vi "template.vi"() -> ()   [LabVIEW 2023]
uses:
  states.ctl
panel:
  in  "Stop Receiving GPS Data":bool
  in  "Stop Receiving Safety Data":bool
  in  "Start":bool
  in  "Stop":bool
  in  "Speed Threshold (km/h)":dbl
  out "Arm System":bool
  out "Laser 2":bool
  out "Laser 1":bool
  out "Safety System 2":bool[](array[boolean])
  out "Safety System 1":bool[](array[boolean])
  out "GPS":cluster{"Lat":dbl, "Lon":dbl, "Speed":dbl} {"Lon" format="%#_15g"; "Lat" format="%#_16g"}
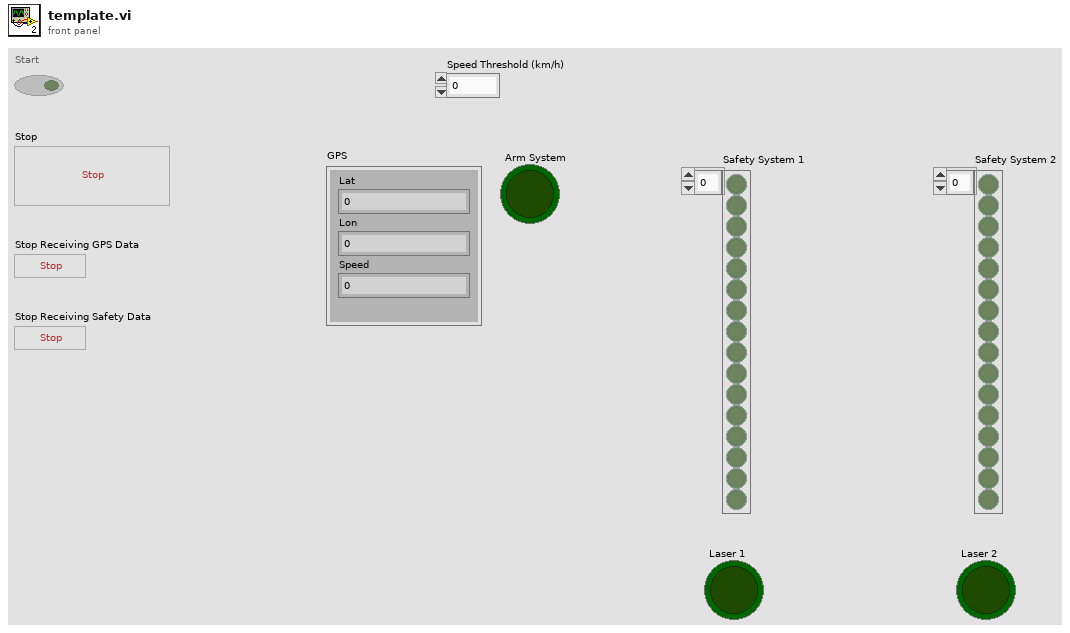
[diagram p1: front panel]
types:
  T1 = typedef "states.ctl" = enum16{"Set Speed Threshold", "Wait for Start", "Wait for TCP", "Main Loop"}
  T2 = enum8{"Enabled", "Disabled", "Disabled and Grayed Out"}
  T3 = enum16{"Standard", "Buffered", "CRLF", "Immediate"}
  T4 = cluster{"Latitude":dbl, "Longitude":dbl, "speed":dbl}
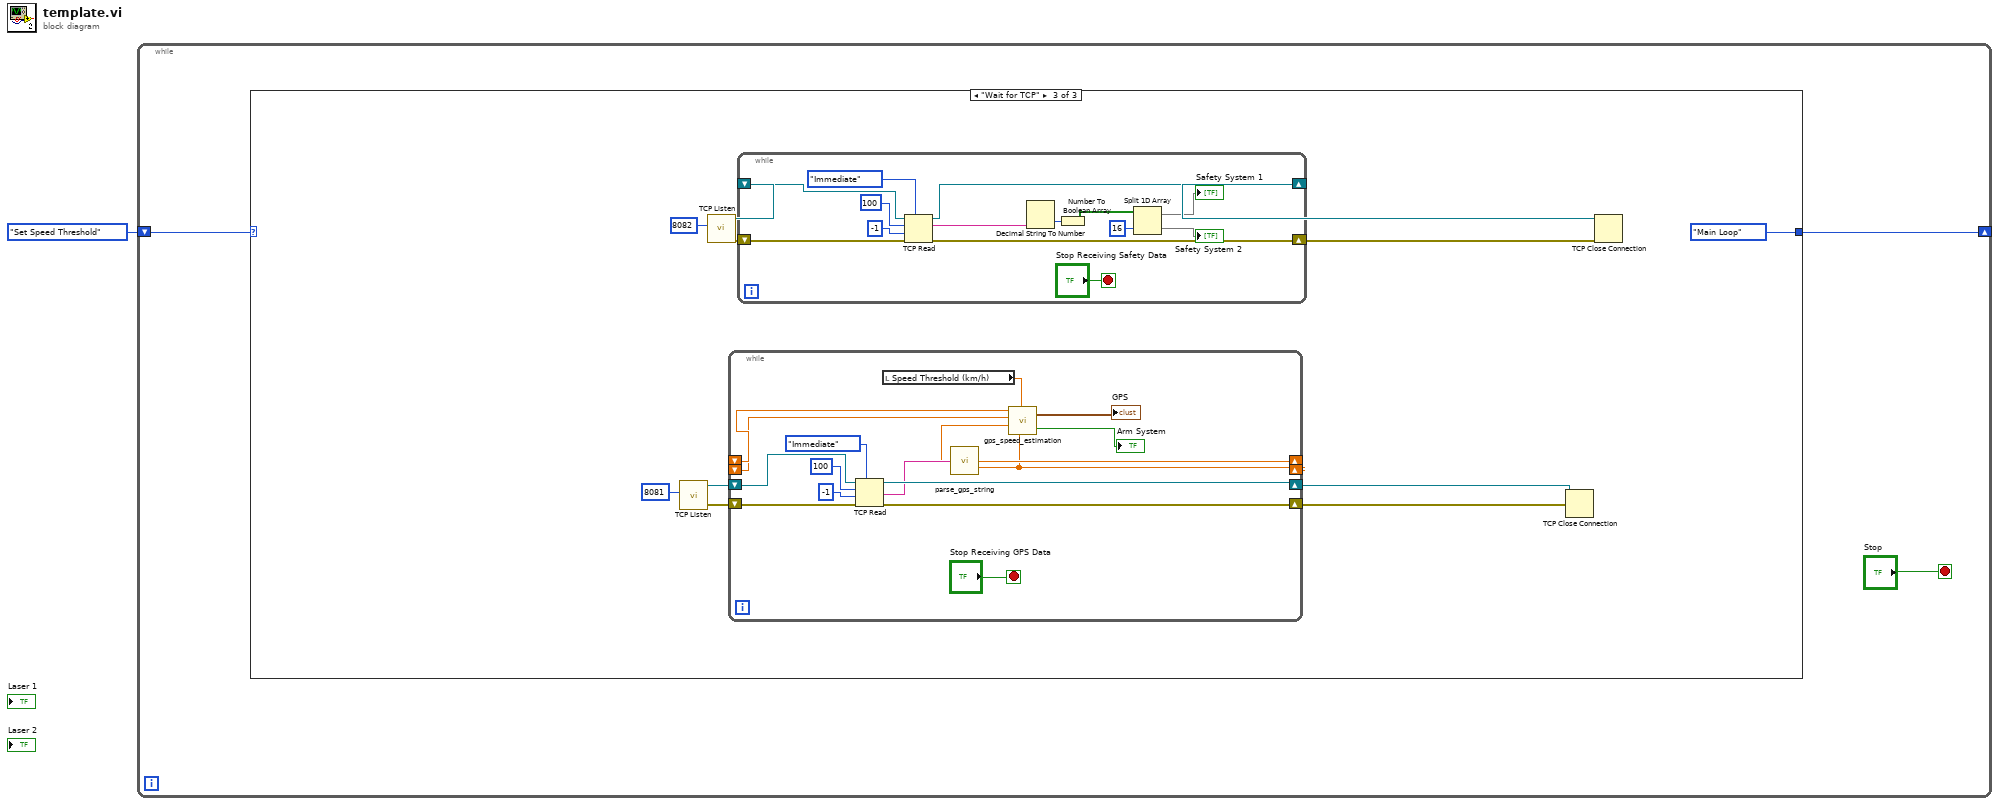
[diagram p0: block diagram]
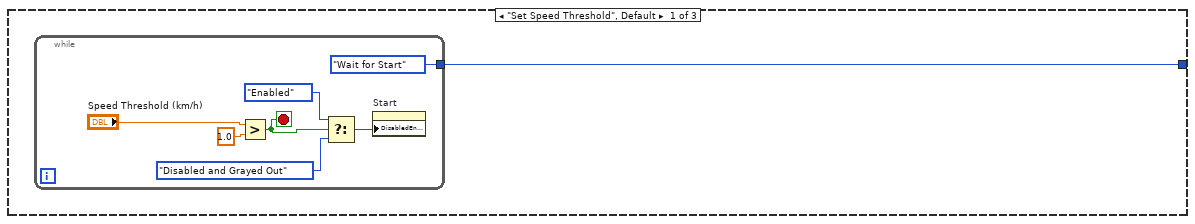
[diagram p2: hidden frame]
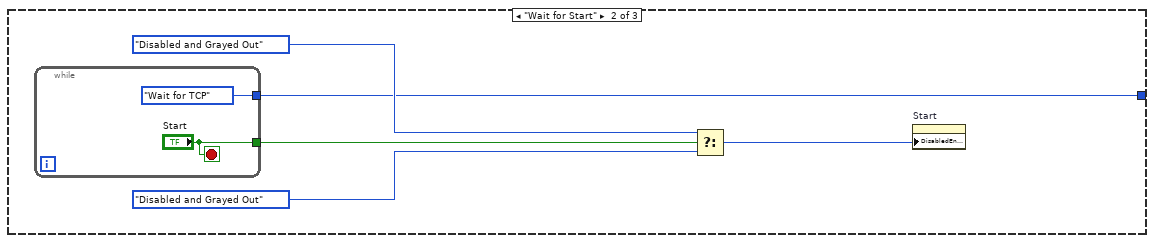
[diagram p3: hidden frame]
diagram:
  n1 = while {
    shift-right: [w2] -> _
    shift-left: states."Set Speed Threshold" -> [w4]
    stop <- "Stop" stop-if-true
    n2 = case shown="\"Wait for TCP\"" w4 {
      tunnel: [w5 w13 states."Main Loop"] -> w2
      frame "Set Speed Threshold", Default {
        n3 = while {
          tunnel: [states."Wait for Start"] -> w5
          stop <- w9 stop-if-true
          n4 = Greater?(x="Speed Threshold (km/h)", y=1.0) -> (0:w9:bool)
          n5 = Select(t=T2."Enabled" ("Disabled"), s=w9, f=T2."Disabled and Grayed Out" ("Disabled")) -> (s? t:f=w10:T2)
          n6 = property on="Start" class="Bool (strict)"("DisabledEnum"=w10) -> ()  [unwired: 2 in, 2 out]
        }
      }
      frame "Wait for Start" {
        n7 = while {
          tunnel: ["Start"] -> w17
          tunnel: [states."Wait for TCP"] -> w13
          stop <- "Start" stop-if-true
        }
        n8 = Select(t=T2."Disabled and Grayed Out" ("Disabled"), s=w17, f=T2."Disabled and Grayed Out" ("Disabled")) -> (s? t:f=w14:T2)
        n9 = property on="Start" class="Bool (strict)"("DisabledEnum"=w14) -> ()  [unwired: 2 in, 2 out]
      }
      frame "Wait for TCP" {
        n10 = call <vilib>:"TCP Listen.vi"("port"=u16 8081) -> ("error out"=w22:errorcluster, "connection ID"=w24:refnum<k5>)  [unwired: 6 in, 3 out]
        n11 = call <vilib>:"TCP Listen.vi"("port"=u16 8082) -> ("error out"=w27:errorcluster, "connection ID"=w29:refnum<k5>)  [unwired: 6 in, 3 out]
        n12 = while {
          shift-right: [w41] -> w23
          shift-left: w24 -> [w44]
          shift-right: [w39] -> w21
          shift-left: w22 -> [w46]
          shift-right: [w34] -> _
          shift-left: _ -> [w37]
          shift-right: [w33] -> _
          shift-left: _ -> [w36]
          stop <- "Stop Receiving GPS Data" stop-if-true
          n13 = TCP Read(connection ID=w44, bytes to read=100, error in (no error)=w46, 7:T3."Immediate" ("mode (standard)"), 9:-1) -> (connection ID out=w41:refnum<k5>, data out=w38:string, error out=w39:errorcluster)
          n14 = local read "Speed Threshold (km/h)"() -> (w32:dbl)
          n15 = call "parse_gps_string.vi"("data in"=w38) -> ("Latitude"=w34:dbl, "Longitude"=w33:dbl)  [unwired: 1 out]
          n16 = call "gps_speed_estimation.vi"("LatitudePrev"=w37, "LongitudePrev"=w36, "Latitude"=w34, "Speed Threshold"=w32, "Longitude"=w33) -> ("GPS"=→"GPS":T4, "Arm System"=→"Arm System":bool)
        }
        n17 = while {
          shift-right: [w55] -> w28
          shift-left: w29 -> [w58]
          shift-right: [w53] -> w26
          shift-left: w27 -> [w60]
          stop <- "Stop Receiving Safety Data" stop-if-true
          n18 = TCP Read(connection ID=w58, bytes to read=100, error in (no error)=w60, 7:T3."Immediate" ("mode (standard)"), 9:-1) -> (connection ID out=w55:refnum<k5>, data out=w51:string, error out=w53:errorcluster)
          n19 = Decimal String To Number(string=w51) -> (number=w52:i32)  [unwired: 2 in, 1 out]
          n20 = Number To Boolean Array(number=w52) -> (Boolean array=w50:bool[])
          n21 = Split 1D Array(array=w50, index=16) -> (first subarray=→"Safety System 1":bool[], second subarray=→"Safety System 2":bool[])
        }
        n22 = TCP Close Connection(connection ID=w23, error in (no error)=w21) -> ()  [unwired: 1 in, 2 out]
        n23 = TCP Close Connection(connection ID=w28, error in (no error)=w26) -> ()  [unwired: 1 in, 2 out]
      }
    }
  }
